vi "Serial Data Communication.vi"() -> ()   [LabVIEW 2020]
uses:
  <vilib>/Instr/_visa.llb/VISA Configure Serial Port (Instr).vi
panel:
  in  "Samples":u16
  out "Waveform Chart":i32(graph)
  in  "Send":bool
  in  "Send":bool
  in  "Channel":u8
  out "Monitor":string
  in  "START":bool
  in  "VISA resource name":refnum<visa-resource-name>
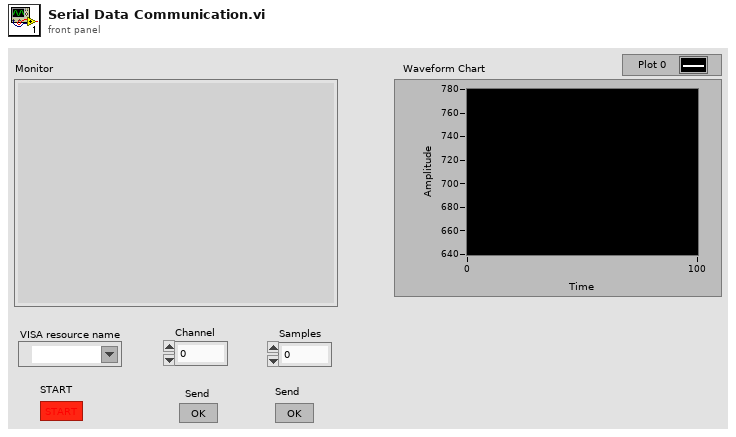
[diagram p1: front panel]
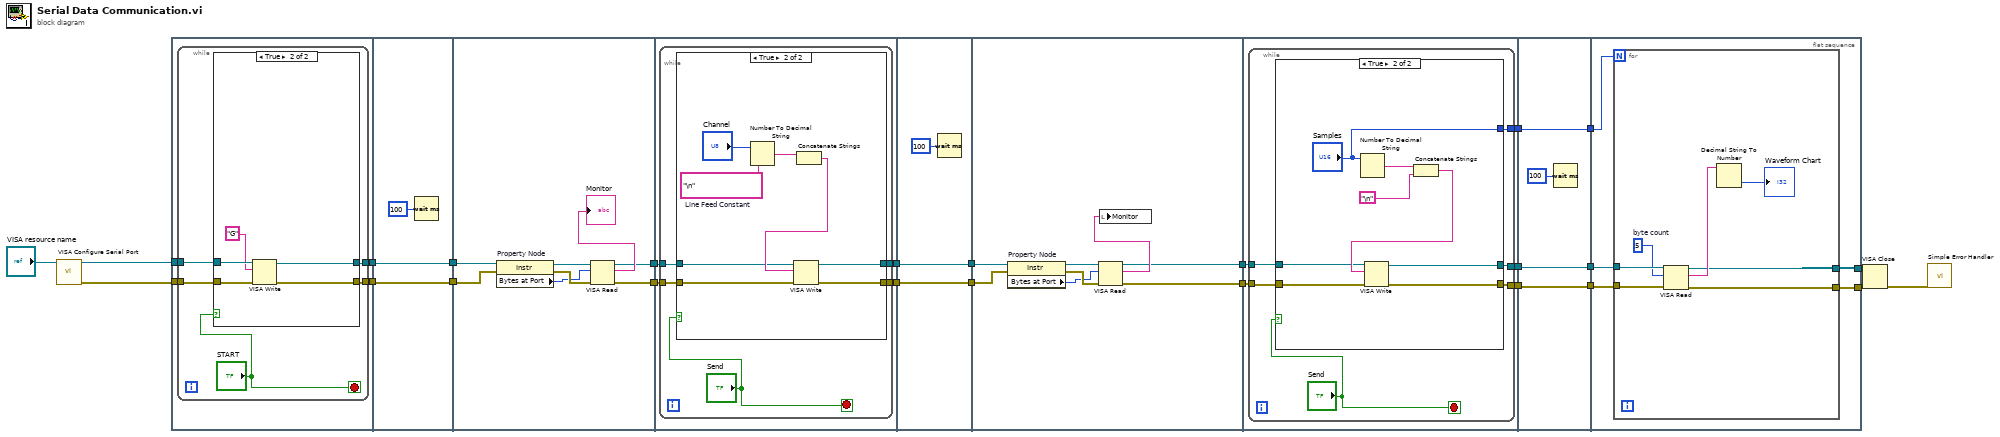
[diagram p0: block diagram]
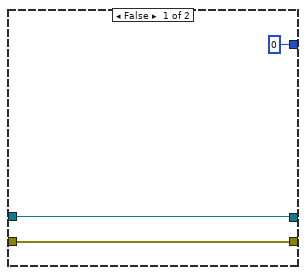
[diagram p4: hidden frame]
diagram:
  n1 = call-poly "VISA Configure Serial Port"("VISA resource name"="VISA resource name") -> ("VISA resource name out"=w23:refnum<visa-resource-name>, "error out"=w22:errorcluster)  [unwired: 13 in]
  n2 = flat-sequence {
    tunnel: w23 -> [w28]
    tunnel: w22 -> [w27]
    tunnel: [w26] -> w20
    tunnel: [w25] -> w18
    tunnel: [w42] -> w21
    tunnel: w20 -> [w42]
    tunnel: [w41] -> w19
    tunnel: w18 -> [w41]
    tunnel: w21 -> [w51]
    tunnel: w19 -> [w50]
    tunnel: [w45] -> w17
    tunnel: [w44] -> w16
    tunnel: w17 -> [w55]
    tunnel: w16 -> [w54]
    tunnel: [w53] -> w14
    tunnel: [w52] -> w12
    tunnel: [w72] -> w15
    tunnel: w14 -> [w72]
    tunnel: [w71] -> w13
    tunnel: w12 -> [w71]
    tunnel: w15 -> [w81]
    tunnel: w13 -> [w80]
    tunnel: [w75] -> w11
    tunnel: [w74] -> w10
    tunnel: w11 -> [w86]
    tunnel: w10 -> [w85]
    tunnel: [w84] -> w9
    tunnel: [w83] -> w6
    tunnel: [w82] -> w4
    tunnel: w9 -> [w106]
    tunnel: [w106] -> w8
    tunnel: [w105] -> w7
    tunnel: w6 -> [w105]
    tunnel: [w104] -> w5
    tunnel: w4 -> [w104]
    tunnel: w8 -> [w112]
    tunnel: w7 -> [w111]
    tunnel: w5 -> [w110]
    tunnel: [w109] -> w3
    tunnel: [w108] -> w2
    frame #0 {
      n3 = while {
        tunnel: w28 -> [w32]
        tunnel: w27 -> [w31]
        tunnel: [w30] -> w26
        tunnel: [w29] -> w25
        stop <- "START" stop-if-true
        n4 = case shown="True" "START" {
          tunnel: w32 -> [w35 w40]
          tunnel: w31 -> [w34 w39]
          tunnel: [w35 w37] -> w30
          tunnel: [w34 w36] -> w29
          frame False {
          }
          frame True {
            n5 = VISA Write(VISA resource name=w40, write buffer="G", error in (no error)=w39) -> (VISA resource name out=w37:refnum<visa-resource-name>, error out=w36:errorcluster)  [unwired: 1 out]
          }
        }
      }
    }
    frame #1 {
      n6 = Wait (ms)(milliseconds to wait=u32 100) -> ()  [unwired: 1 out]
    }
    frame #2 {
      n7 = property on="Property Node" class="Instr"(reference=w51, error in=w50) -> (reference out=w49:refnum<visa-resource-name>, error out=w48:errorcluster, "Bytes at Port"=w47:u32)
      n8 = VISA Read(VISA resource name=w49, byte count=w47, error in (no error)=w48) -> (VISA resource name out=w45:refnum<visa-resource-name>, read buffer=→"Monitor":string, error out=w44:errorcluster)  [unwired: 1 out]
    }
    frame #3 {
      n9 = while {
        tunnel: w55 -> [w59]
        tunnel: w54 -> [w58]
        tunnel: [w57] -> w53
        tunnel: [w56] -> w52
        stop <- "Send" stop-if-true
        n10 = case shown="True" "Send" {
          tunnel: w59 -> [w62 w66]
          tunnel: w58 -> [w61 w65]
          tunnel: [w62 w64] -> w57
          tunnel: [w61 w63] -> w56
          frame False {
          }
          frame True {
            w68 = "\n"  # Line Feed Constant
            n11 = Number To Decimal String(number="Channel") -> (decimal integer string=w69:string)  [unwired: 1 in]
            n12 = Concatenate Strings "Concatenate Strings"(w69, w68) -> (w67:string)
            n13 = VISA Write(VISA resource name=w66, write buffer=w67, error in (no error)=w65) -> (VISA resource name out=w64:refnum<visa-resource-name>, error out=w63:errorcluster)  [unwired: 1 out]
          }
        }
      }
    }
    frame #4 {
      n14 = Wait (ms)(milliseconds to wait=u32 100) -> ()  [unwired: 1 out]
    }
    frame #5 {
      n15 = property on="Property Node" class="Instr"(reference=w81, error in=w80) -> (reference out=w77:refnum<visa-resource-name>, error out=w79:errorcluster, "Bytes at Port"=w78:u32)
      n16 = VISA Read(VISA resource name=w77, byte count=w78, error in (no error)=w79) -> (VISA resource name out=w75:refnum<visa-resource-name>, read buffer=w76:string, error out=w74:errorcluster)  [unwired: 1 out]
      n17 = local write "Monitor"(w76) -> ()
    }
    frame #6 {
      n18 = while {
        tunnel: w86 -> [w91]
        tunnel: w85 -> [w90]
        tunnel: [w87] -> w84
        tunnel: [w89] -> w83
        tunnel: [w88] -> w82
        stop <- "Send" stop-if-true
        n19 = case shown="True" "Send" {
          tunnel: w91 -> [w95 w100]
          tunnel: w90 -> [w94 w99]
          tunnel: [w95 w98] -> w89
          tunnel: [w94 w97] -> w88
          tunnel: [u16 0 ("Samples") "Samples"] -> w87
          frame False {
          }
          frame True {
            n20 = Number To Decimal String(number="Samples") -> (decimal integer string=w102:string)  [unwired: 1 in]
            n21 = Concatenate Strings "Concatenate Strings"(w102, "\n") -> (w103:string)
            n22 = VISA Write(VISA resource name=w100, write buffer=w103, error in (no error)=w99) -> (VISA resource name out=w98:refnum<visa-resource-name>, error out=w97:errorcluster)  [unwired: 1 out]
          }
        }
      }
    }
    frame #7 {
      n23 = Wait (ms)(milliseconds to wait=u32 100) -> ()  [unwired: 1 out]
    }
    frame #8 {
      n24 = for {
        N: w112 -> [_]
        tunnel: w111 -> [w119]
        tunnel: w110 -> [w118]
        tunnel: [w114] -> w109
        tunnel: [w113] -> w108
        w117 = u32 5  # byte count
        n25 = VISA Read(VISA resource name=w119, byte count=w117, error in (no error)=w118) -> (VISA resource name out=w114:refnum<visa-resource-name>, read buffer=w116:string, error out=w113:errorcluster)  [unwired: 1 out]
        n26 = Decimal String To Number(string=w116) -> (number=→"Waveform Chart":i32)  [unwired: 2 in, 1 out]
      }
    }
  }
  n27 = VISA Close(VISA resource name=w3, error in (no error)=w2) -> (error out=w1:errorcluster)
  n28 = call <vilib>:"Simple Error Handler.vi"("error in (no error)"=w1) -> ()  [unwired: 4 in, 5 out]
